vi "getcmd.vi"(8 "error in (no error)":errorcluster, 11 "String":string) -> (0 "error IO":errorcluster, 2 "CMD":cluster{T1})   [LabVIEW 2016]
uses:
  typedefs/commands.ctl
  typedefs/commandtypes.ctl
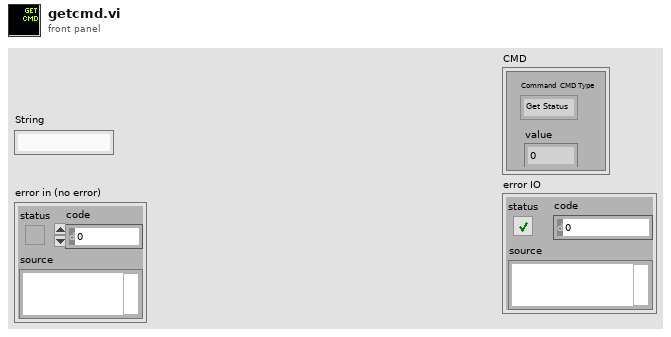
[diagram p1: front panel]
types:
  T1 = typedef "commands.ctl" = cluster{"Command  CMD Type":T2, "value":dbl}
  T2 = typedef "commandtypes.ctl" = enum16{"Get Status", "Setpoint", "Ramp rate", "Pause", "Ramp up"}
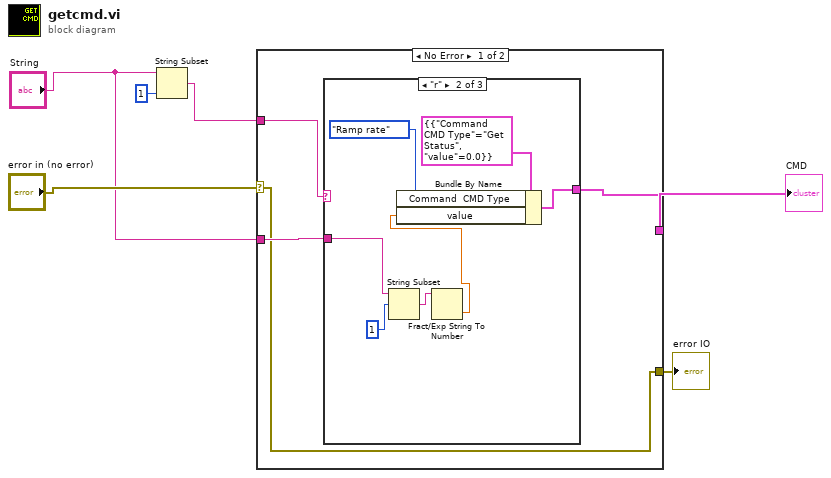
[diagram p0: block diagram]
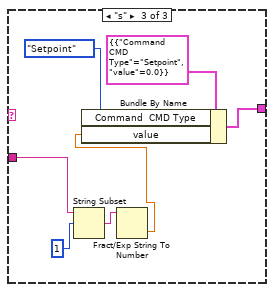
[diagram p3: hidden frame]
diagram:
  n1 = String Subset(string="String", length (rest)=1 ("length (rest)")) -> (substring=w4:string)  [unwired: 1 in]
  n2 = case shown="No Error" "error in (no error)" {
    selector: "error in (no error)" -> [w7 w25]
    tunnel: w4 -> [w10 _]
    tunnel: "String" -> [w9 _]
    tunnel: [w8 _] -> w2
    tunnel: [w7 w25] -> w1
    frame No Error {
      n3 = case shown="\"r\"" w10 {
        tunnel: w9 -> [_ w17 w24]
        tunnel: [_ w14 w21] -> w8
        frame "False", Default {
        }
        frame "r" {
          n4 = String Subset(string=w17, offset (0)=1) -> (substring=w15:string)  [unwired: 1 in]
          n5 = Fract/Exp String To Number(string=w15) -> (number=w11:dbl)  [unwired: 3 in, 1 out]
          n6 = Bundle By Name(cluster=cluster{T1} {{"Command  CMD Type"=enum."Get Status", "value"=0.0}} ("input cluster"), "Command  CMD Type"=commandtypes."Ramp rate" (".Command  CMD Type"), "value"=w11) -> (w14:cluster{T1})
        }
        frame "s" {
          n7 = String Subset(string=w24, offset (0)=1) -> (substring=w22:string)  [unwired: 1 in]
          n8 = Fract/Exp String To Number(string=w22) -> (number=w18:dbl)  [unwired: 3 in, 1 out]
          n9 = Bundle By Name(cluster=cluster{T1} {{"Command  CMD Type"=enum."Setpoint", "value"=0.0}} ("input cluster"), "Command  CMD Type"=commandtypes."Setpoint" (".Command  CMD Type"), "value"=w18) -> (w21:cluster{T1})
        }
      }
    }
    frame Error {
    }
  }
  "CMD" <- w2
  "error IO" <- w1
